vi "Delete Notification From Map.vi"(7 "Alias":string, 8 "error in (no error)":errorcluster, 10 "Symbol Name":string, 11 "TwinCAT ADS in":refnum<class "TwinCAT ADS.lvclass">) -> (0 "error out":errorcluster, 3 "TwinCAT ADS out":refnum<class "TwinCAT ADS.lvclass">)   [LabVIEW 2018, in "TwinCAT ADS.lvclass"]
uses:
  TwinCAT ADS.lvclass
  TwinCAT ADS.lvclass/TwinCAT ADS.ctl
  Controls/Notifcation Map Value.ctl
  <vilib>/Utility/error.llb/Trim Whitespace.vi
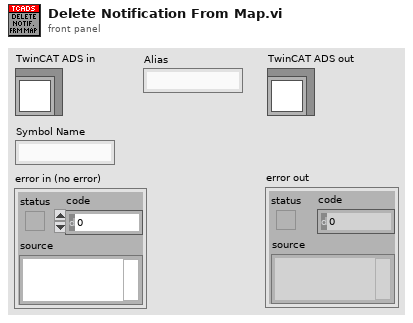
[diagram p1: front panel]
types:
  T1 = typedef "TwinCAT ADS.lvclass/Notifcation Map Value.ctl" = cluster{"Handle":i32, "Cycle Time":i32}
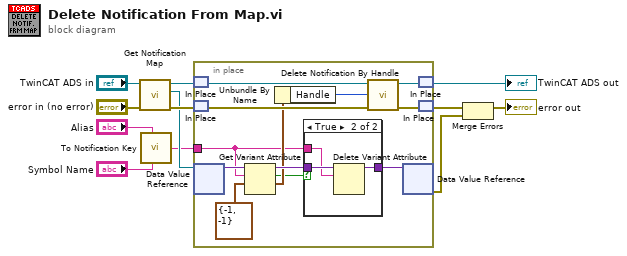
[diagram p0: block diagram]
diagram:
  n1 = call "Get Notification Map.vi"("error in (no error)"="error in (no error)", "TwinCAT ADS in"="TwinCAT ADS in") -> ("error out"=w9:errorcluster, "Notification Map"=w5:refnum<data-value>, "TwinCAT ADS out"=w10:refnum<class "TwinCAT ADS.lvclass">)  [unwired: 7 in]
  n2 = call "To Notification Key.vi"("Alias"="Alias", "Symbol Name"="Symbol Name") -> ("Key"=w3:string)  [unwired: 5 in]
  n3 = in-place {
    in-place-border: w3 -> [w13]
    n4 = in-place-match #1(w10) -> (w20:refnum<class "TwinCAT ADS.lvclass">)
    n5 = in-place-match #2(w9) -> (w21:errorcluster)
    n6 = in-place-dvr #3(w5) -> (w22:variant)  [unwired: 1 out]
    n7 = Get Variant Attribute(Variant=w22, name=w13, default value (empty Variant)=T1 {"Handle"=-1, "Cycle Time"=-1} ("Value")) -> (duplicate Variant=w18:variant, found=w16:bool, value=w17:T1)  [unwired: 1 in, 1 out]
    n8 = Unbundle By Name(w17) -> ("Handle"=w19:i32)
    n9 = case shown="True" w16 {
      tunnel: [w25 w28] -> w24
      tunnel: w18 -> [w25 w27]
      tunnel: w13 -> [_ w26]
      frame False {
      }
      frame True {
        n10 = Delete Variant Attribute(6:w26, 7:w27) -> (3:w28:variant)  [unwired: 1 in, 2 out]
      }
    }
    n11 = call "Delete Notification By Handle.vi"("error in (no error)"=w21, "Handle"=w19, "TwinCAT ADS in"=w20) -> ("error out"=w14:errorcluster, "TwinCAT ADS out"=w15:refnum<class "TwinCAT ADS.lvclass">)  [unwired: 7 in]
    n12 = in-place-dvr #3(w24) -> (w12:errorcluster)  [unwired: 1 out]
    n13 = in-place-match #1(w15) -> (→"TwinCAT ADS out":refnum<class "TwinCAT ADS.lvclass">)
    n14 = in-place-match #2(w14) -> (w2:errorcluster)
  }
  n15 = Merge Errors(w2, w12) -> (→"error out":errorcluster)
